vi "XLP80_HH_Close.vi"(8 "err in":errorcluster) -> (0 "err out":errorcluster)   [LabVIEW 2021]
uses:
  XLP80_Globals/Globals_Settings_XLP80.vi
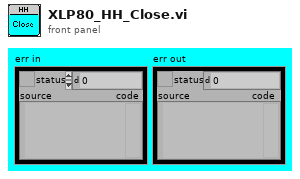
[diagram p1: front panel]
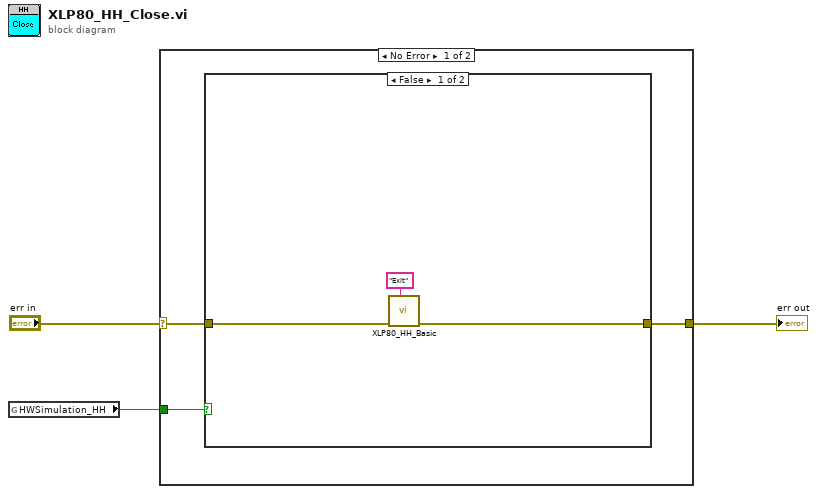
[diagram p0: block diagram]
diagram:
  n1 = global read "Globals_Settings_XLP80.vi" "HWSimulation_HH"() -> (w1:bool)
  n2 = case shown="No Error" "err in" {
    selector: "err in" -> [w6 w11]
    tunnel: [w4 w11] -> w2
    tunnel: w1 -> [w5 _]
    frame No Error {
      n3 = case shown="False" w5 {
        tunnel: w6 -> [w8 w10]
        tunnel: [w7 w10] -> w4
        frame False {
          n4 = call "XLP80_HH_Basic.vi"("Function"="Exit", "err in"=w8) -> ("err out"=w7:errorcluster)  [unwired: 9 in]
        }
        frame True {
        }
      }
    }
    frame Error {
    }
  }
  "err out" <- w2
